vi "Load Help File.vi"(8 "error in (no error)":errorcluster, 9 "HTML File":string="MainPage_J1939.html", 10 "Main CHM File":string="J1939.chm", 11 "SHDocVw.IWebBrowser2":refnum<k7>(container)) -> (0 "error out":errorcluster)   [LabVIEW 2018, in "Instrument Addon System Explorer.lvlib"]
uses:
  Instrument Addon System Explorer.lvlib
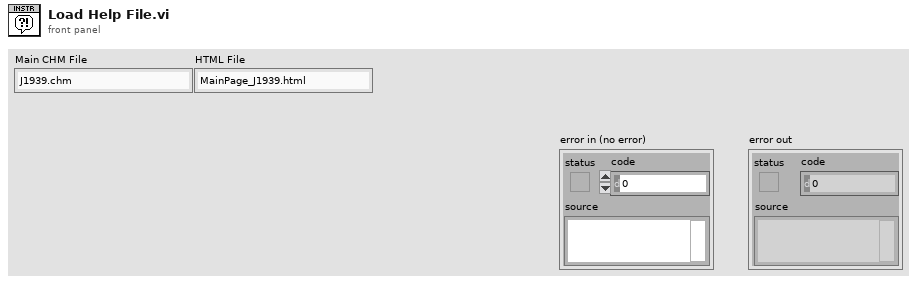
[diagram p1: front panel]
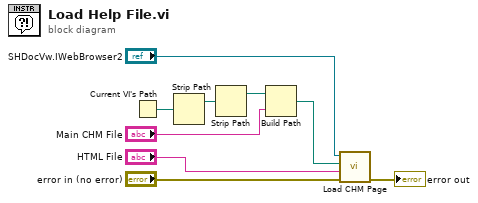
[diagram p0: block diagram]
diagram:
  n1 = Current VI's Path() -> (path=w9:path)
  n2 = Strip Path(path=w9) -> (stripped path=w8:path)  [unwired: 1 out]
  n3 = Strip Path(path=w8) -> (stripped path=w7:path)  [unwired: 1 out]
  n4 = Build Path(base path=w7, name or relative path="Main CHM File") -> (appended path=w6:path)
  n5 = call <vilib>:"Load CHM Page.vi"("error in (no error)"="error in (no error)", "HTML File"="HTML File", "Compiled CHM Path"=w6, "Web Browser Reference"="SHDocVw.IWebBrowser2") -> ("error out"=→"error out":errorcluster)  [unwired: 7 in]
